vi "Write Launch Guest Manager Msg.vi"(10 "Rooms Manager UI.lvlib:Launch Guest Manager Msg.lvclass":refnum<class "Launch Guest Manager Msg.lvclass">, 11 "Rooms Manager UI in":refnum<class "Rooms Manager UI.lvclass">) -> (3 "Rooms Manager UI out":refnum<class "Rooms Manager UI.lvclass">)   [LabVIEW 2023, in "Rooms Manager UI.lvlib" / "Rooms Manager UI.lvclass"]
uses:
  Rooms Manager UI.lvclass
  Rooms Manager UI Messages/Launch Guest Manager Msg/Launch Guest Manager Msg.lvclass
  Rooms Manager UI.lvclass/Rooms Manager UI.ctl
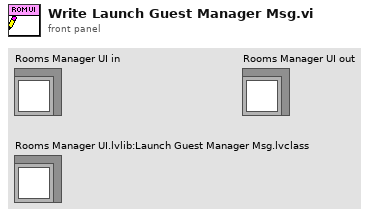
[diagram p1: front panel]
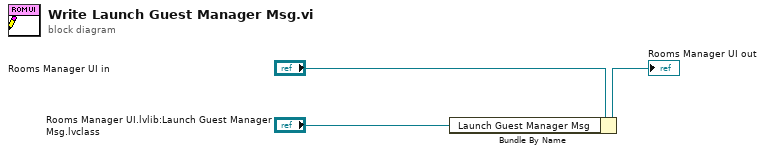
[diagram p0: block diagram]
diagram:
  n1 = Bundle By Name(cluster="Rooms Manager UI in", "Launch Guest Manager Msg"="Rooms Manager UI.lvlib:Launch Guest Manager Msg.lvclass") -> (→"Rooms Manager UI out":refnum<class "Rooms Manager UI.lvclass">)
